vi "FGV Change laser wavelength.vi"(7 "FGV Actions":enum16{"Get", "Set"}(ring), 8 "error in (no error)":errorcluster, 10 "Wavelength IN":i16, 11 "Change Wavelength ? IN":bool) -> (0 "error out":errorcluster, 2 "Wavelength OUT":i16, 3 "Change Wavelength ? OUT":bool)   [LabVIEW 2017]
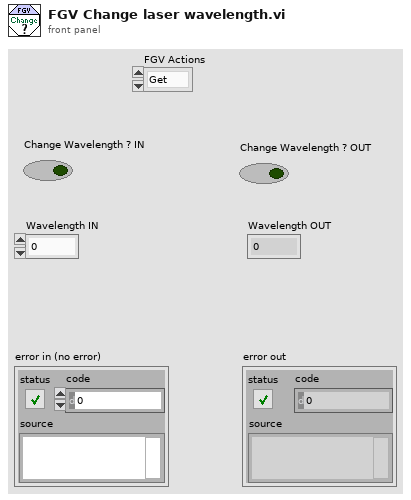
[diagram p1: front panel]
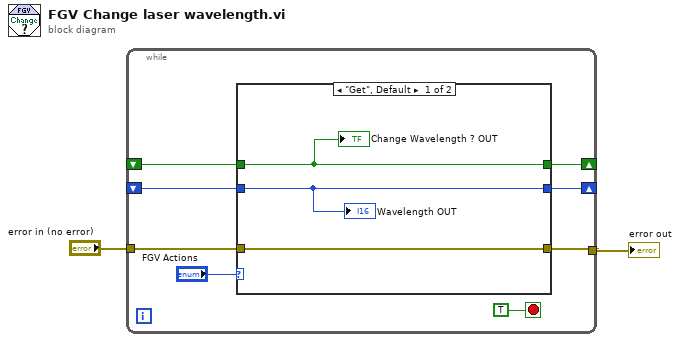
[diagram p0: block diagram]
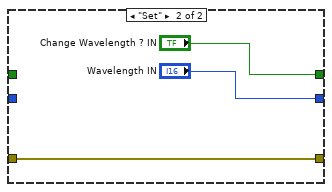
[diagram p2: hidden frame]
diagram:
  n1 = while {
    shift-right: [w8] -> _
    shift-left: _ -> [w7]
    tunnel: "error in (no error)" -> [w6]
    tunnel: [w5] -> w1
    shift-right: [w4] -> _
    shift-left: _ -> [w3]
    stop <- TRUE stop-if-true
    n2 = case shown="\"Get\", Default" "FGV Actions" {
      tunnel: [w12 "Change Wavelength ? IN"] -> w8
      tunnel: w7 -> [w12 _]
      tunnel: w6 -> [w13 w16]
      tunnel: [w13 w16] -> w5
      tunnel: [w11 "Wavelength IN"] -> w4
      tunnel: w3 -> [w11 _]
      frame "Get", Default {
        "Change Wavelength ? OUT" <- w12
        "Wavelength OUT" <- w11
      }
      frame "Set" {
      }
    }
  }
  "error out" <- w1
